vi "A170316-11_config.vi"() -> ()   [LabVIEW 2020]
uses:
  Global_Variable/Global.vi
  Database/Global1.vi
  <vilib>/Utility/config.llb/NI_LVConfig.lvlib
panel:
  in  "选项卡控件":enum32{"检具参数", "备用参数", "产品管理"}(tab)
  in  "检具选择":bool[](array[boolean])
  in  "删除":bool
  in  "确定":bool
  in  "添加":bool
  in  "退出":bool
  in  "更新":bool
  in  "产品型号":string(combo)
  in  "请输入添加的产品名称":string
  in  "请选择要删除的产品":string(combo)
  # "总成检验"
  # "检具1"
  # "检具2"
  # "检具3"
  # "检具4"
  # "检具5"
  # "检具6"
  # "检具7"
  # "检具8"
  # "检具9"
  # "检具10"
  # "检具11"
  # "检具12"
  # "检具13"
  # "检具14"
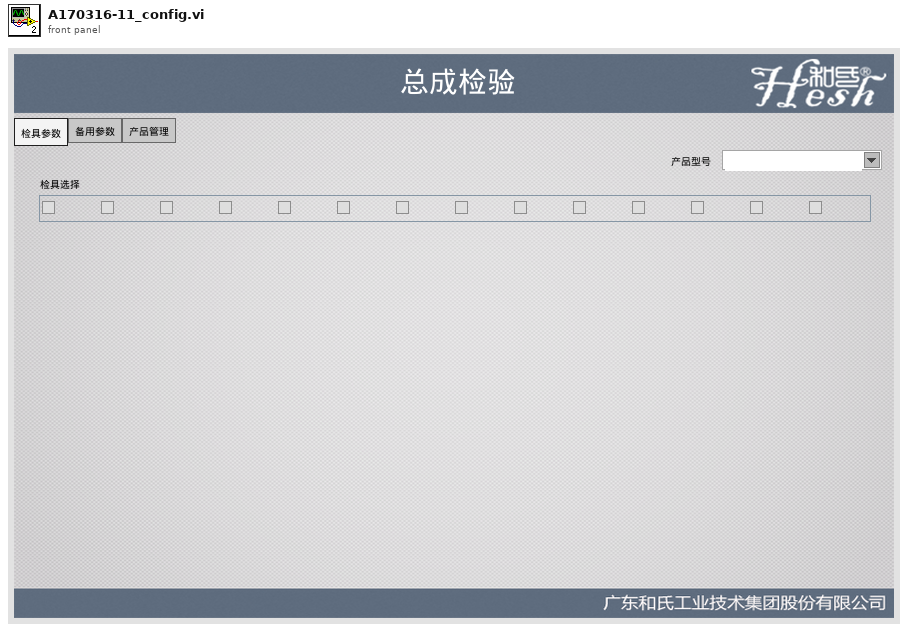
[diagram p1: front panel]
types:
  T1 = typedef "NI_LVConfig.lvlib/Config Data RefNum.ctl" = refnum<k1>
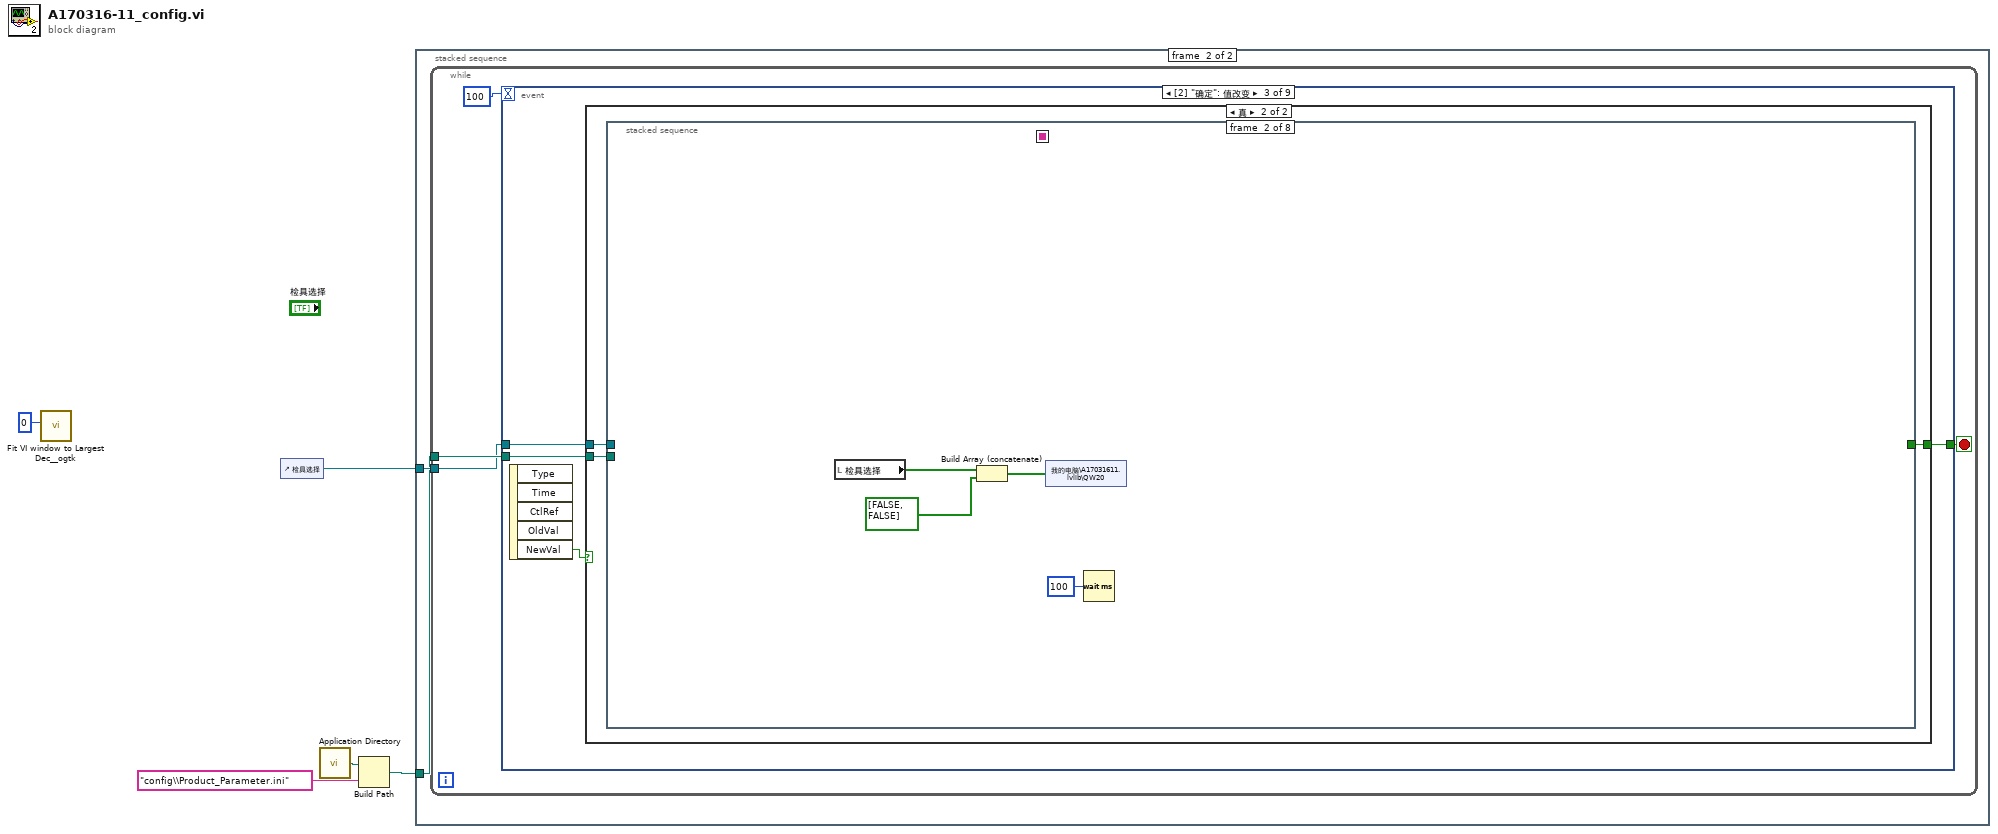
[diagram p0: block diagram]
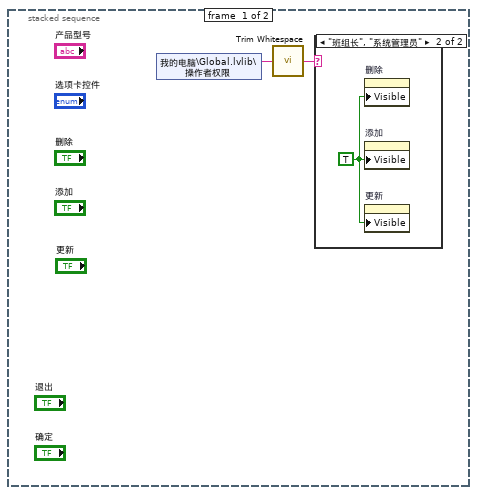
[diagram p2: hidden frame]
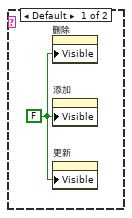
[diagram p3: hidden frame]
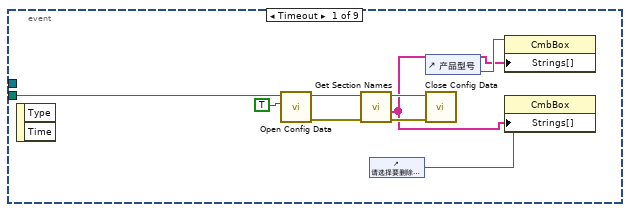
[diagram p4: hidden frame]
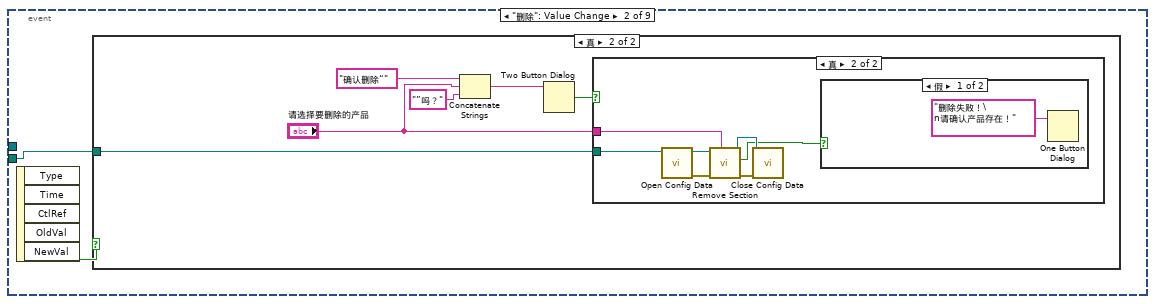
[diagram p5: hidden frame]
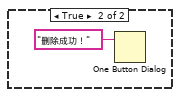
[diagram p8: hidden frame]
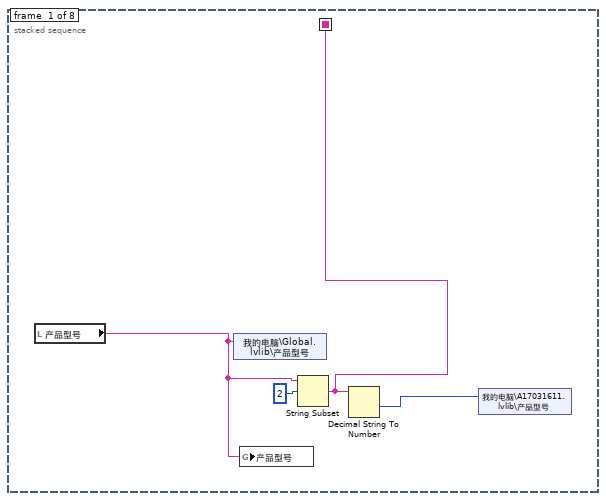
[diagram p10: hidden frame]
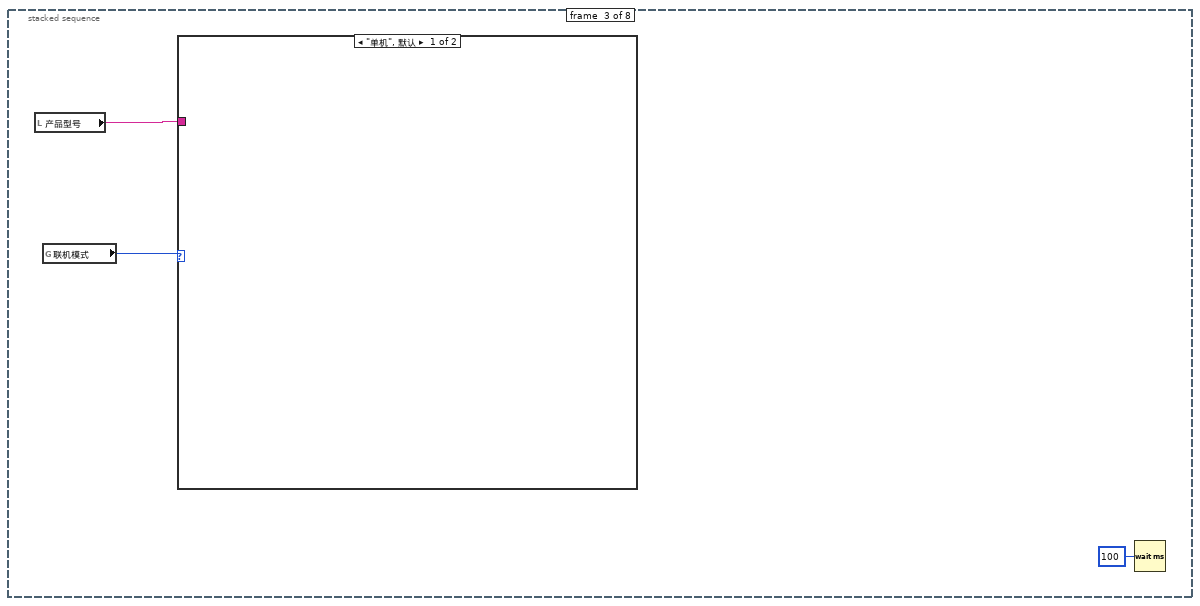
[diagram p11: hidden frame]
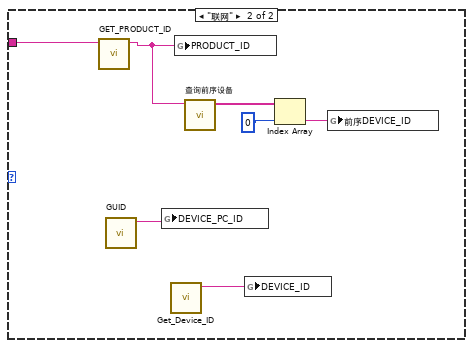
[diagram p12: hidden frame]
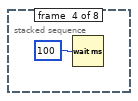
[diagram p13: hidden frame]
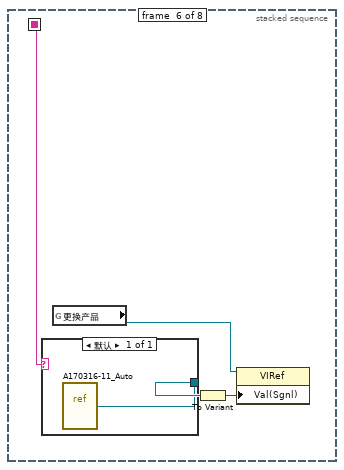
[diagram p15: hidden frame]
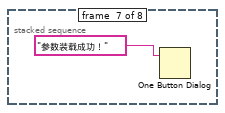
[diagram p16: hidden frame]
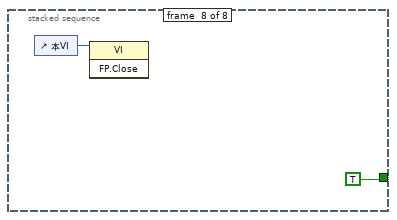
[diagram p17: hidden frame]
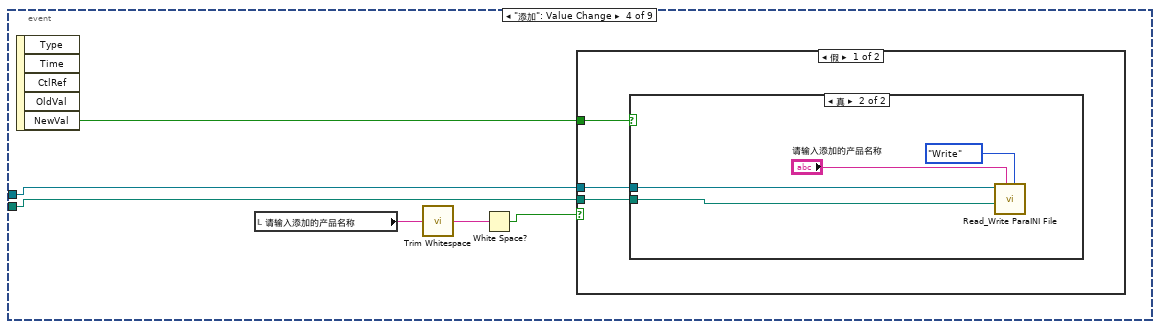
[diagram p18: hidden frame]
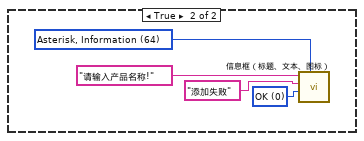
[diagram p20: hidden frame]
diagram:
  n1 = call <userlib>:"Fit VI window to Largest Dec__ogtk.vi"("border spacing (2 px)"=0) -> ()  [unwired: 5 in, 2 out]
  n2 = control-ref of="检具选择"() -> (w1:refnum<vi>)
  n3 = call <vilib>:"Application Directory.vi"() -> ("Application Directory"=w5:path)
  n4 = Build Path(base path=w5, name or relative path="config\\Product_Parameter.ini" ("名称或相对路径")) -> (appended path=w3:path)
  n5 = stacked-sequence {
    tunnel: w1 -> [_ w11]
    tunnel: w3 -> [_ w10]
    frame #0 {
      n6 = shared-variable "我的电脑\\Global.lvlib\\操作者权限"() -> (w7:string)  [unwired: 1 in, 1 out]
      n7 = call <vilib>:"Trim Whitespace.vi"("string"=w7) -> ("trimmed string"=w6:string)  [unwired: 1 in]
      n8 = case shown="\"班组长\", \"系统管理员\"" w6 {
        frame Default {
          w8 = FALSE ("可见")
          n9 = property on="删除" class="Bool (严格)"("Visible"=w8) -> ()  [unwired: 2 in, 2 out]
          n10 = property on="添加" class="Bool (严格)"("Visible"=w8) -> ()  [unwired: 2 in, 2 out]
          n11 = property on="更新" class="Bool (严格)"("Visible"=w8) -> ()  [unwired: 2 in, 2 out]
        }
        frame "班组长", "系统管理员" {
          w9 = TRUE ("可见")
          n12 = property on="删除" class="Bool (严格)"("Visible"=w9) -> ()  [unwired: 2 in, 2 out]
          n13 = property on="添加" class="Bool (严格)"("Visible"=w9) -> ()  [unwired: 2 in, 2 out]
          n14 = property on="更新" class="Bool (严格)"("Visible"=w9) -> ()  [unwired: 2 in, 2 out]
        }
      }
    }
    frame #1 {
      n15 = while {
        tunnel: w10 -> [w15]
        tunnel: w11 -> [w13]
        stop <- w14 stop-if-true
        n16 = event shown="[2] \"确定\": 值改变" {
          selector: _ -> [_ _ _ _ _ _ _ _ _]
          dyn-events: _ -> [_ _ _ _ _ _ _ _ _]
          timeout: 100 -> [_ _ _ _ _ _ _ _ _]
          tunnel: w15 -> [w19 w26 w42 w80 w95 _ w112 _ _]
          tunnel: [_ _ w44 _ _ TRUE _ _ TRUE] -> w14
          tunnel: w13 -> [_ _ w43 w81 w96 _ w111 _ _]
          event Timeout {
            n17 = event-data() -> ()  [unwired: 1 in, 2 out]
            n18 = call <vilib>:"Open Config Data.vi"("create file if necessary (T)"=TRUE, "configuration file path"=w19) -> ("error out"=w21:errorcluster, "refnum"=w20:T1)  [unwired: 7 in, 1 out]
            n19 = call <vilib>:"Get Section Names.vi"("error in (no error)"=w21, "refnum"=w20) -> ("error out"=w23:errorcluster, "section names"=w16:string[], "refnum out"=w22:T1)  [unwired: 7 in]
            n20 = control-ref of="请选择要删除的产品"() -> (w17:refnum<vi>)
            n21 = control-ref of="产品型号"() -> (w18:refnum<vi>)
            n22 = call <vilib>:"Close Config Data.vi"("error in (no error)"=w23, "refnum"=w22) -> ()  [unwired: 8 in, 2 out]
            n23 = property on="属性节点" class="CmbBox"(reference=w18, "Strings[]"=w16) -> ()  [unwired: 1 in, 2 out]
            n24 = property on="属性节点" class="CmbBox"(reference=w17, "Strings[]"=w16) -> ()  [unwired: 1 in, 2 out]
          }
          event "删除": Value Change {
            n25 = event-data() -> ("NewVal"=w25:bool)  [unwired: 1 in, 4 out]
            n26 = case shown="真" w25 {
              tunnel: w26 -> [_ w28]
              frame False {
              }
              frame True {
                n27 = Concatenate Strings("确认删除“", "请选择要删除的产品", "”吗？") -> (w30:string)
                n28 = Two Button Dialog(message=w30) -> (T button?=w29:bool)  [unwired: 2 in]
                n29 = case shown="真" w29 {
                  tunnel: w28 -> [_ w34]
                  tunnel: "请选择要删除的产品" -> [_ w33]
                  frame False {
                  }
                  frame True {
                    n30 = call <vilib>:"Open Config Data.vi"("configuration file path"=w34) -> ("error out"=w36:errorcluster, "refnum"=w39:T1)  [unwired: 8 in, 1 out]
                    n31 = call <vilib>:"Remove Section.vi"("section"=w33, "error in (no error)"=w36, "refnum"=w39) -> ("error out"=w38:errorcluster, "section exists?"=w35:bool, "refnum out"=w37:T1)  [unwired: 6 in]
                    n32 = call <vilib>:"Close Config Data.vi"("error in (no error)"=w38, "refnum"=w37) -> ()  [unwired: 8 in, 2 out]
                    n33 = case shown="假" w35 {
                      frame False {
                        n34 = One Button Dialog(message="删除失败！\n请确认产品存在！" ("消息")) -> ()  [unwired: 1 in, 1 out]
                      }
                      frame True {
                        n35 = One Button Dialog(message="删除成功！" ("消息")) -> ()  [unwired: 1 in, 1 out]
                      }
                    }
                  }
                }
              }
            }
          }
          event "确定": Value Change {
            n36 = event-data() -> ("NewVal"=w45:bool)  [unwired: 1 in, 4 out]
            n37 = case shown="真" w45 {
              tunnel: [_ w48] -> w44
              tunnel: w43 -> [_ w47]
              tunnel: w42 -> [_ w46]
              frame False {
              }
              frame True {
                n38 = stacked-sequence {
                  seq-local: [w52 _ _ _ _ _ _ _] -> [_ _ _ _ _ w71 _ _]
                  tunnel: [_ _ _ _ _ _ _ TRUE] -> w48
                  tunnel: w47 -> [_ _ _ _ _ _ _ _]
                  tunnel: w46 -> [_ _ _ _ _ _ _ _]
                  frame #0 {
                    n39 = local read "产品型号"() -> (w49:string)
                    n40 = shared-variable "我的电脑\\Global.lvlib\\产品型号"(w49) -> ()  [unwired: 1 in, 1 out]
                    n41 = global write "Global.vi" "产品型号"(w49) -> ()
                    n42 = String Subset(string=w49, offset (0)=u16 2 ("偏移量(0)")) -> (substring=w52:string)  [unwired: 1 in]
                    n43 = Decimal String To Number(string=w52) -> (number=w50:i32)  [unwired: 2 in, 1 out]
                    n44 = shared-variable "我的电脑\\A17031611.lvlib\\产品型号"(w50) -> ()  [unwired: 1 in, 1 out]
                  }
                  frame #1 {
                    n45 = local read "检具选择"() -> (w55:bool[])
                    n46 = Build Array (concatenate)(w55, bool[] [FALSE, FALSE] ("数组")) -> (w54:bool[])
                    n47 = shared-variable "我的电脑\\A17031611.lvlib\\QW20"(w54) -> ()  [unwired: 1 in, 1 out]
                    n48 = Wait (ms)(milliseconds to wait=u32 100) -> ()  [unwired: 1 out]
                  }
                  frame #2 {
                    n49 = local read "产品型号"() -> (w58:string)
                    n50 = global read "Global1.vi" "联机模式"() -> (w57:enum16{"单机", "联网"})
                    n51 = case shown="\"单机\", 默认" w57 {
                      tunnel: w58 -> [_ w60]
                      frame "单机", Default {
                      }
                      frame "联网" {
                        n52 = call "GET_PRODUCT_ID.vi"("PRODFUCT_NAME"=w60) -> ("PRODUCT_ID"=w65:string)  [unwired: 10 in]
                        n53 = call "GUID.vi"() -> ("trimmed string"=w66:string)  [unwired: 11 in]
                        n54 = global write "Global1.vi" "DEVICE_PC_ID"(w66) -> ()
                        n55 = call "Get_Device_ID.vi"() -> ("Device_ID"=w61:string)  [unwired: 10 in, 1 out]
                        n56 = global write "Global1.vi" "PRODUCT_ID"(w65) -> ()
                        n57 = call "查询前序设备.vi"("PRODUCT_ID"=w65) -> ("前序工位"=w64:string[])  [unwired: 10 in]
                        n58 = global write "Global1.vi" "DEVICE_ID"(w61) -> ()
                        n59 = Index Array(array=w64, index=0 ("索引")) -> (element=w62:string)
                        n60 = global write "Global1.vi" "前序DEVICE_ID"(w62) -> ()
                      }
                    }
                    n61 = Wait (ms)(milliseconds to wait=u32 100) -> ()  [unwired: 1 out]
                  }
                  frame #3 {
                    n62 = Wait (ms)(milliseconds to wait=u32 100) -> ()  [unwired: 1 out]
                  }
                  frame #4 {
                  }
                  frame #5 {
                    n63 = case shown="默认" w71 {
                      tunnel: [w72] -> w68
                      frame 默认 {
                        n64 = vi-ref "A170316-11_Auto.vi"() -> (w72:refnum<vi>)
                      }
                    }
                    n65 = global read "Global.vi" "更换产品"() -> (w70:refnum<vi>)
                    n66 = To Variant(anything=w68) -> (Variant=w69:variant)
                    n67 = property class="VIRef"(reference=w70, "Val(Sgnl)"=w69) -> ()  [unwired: 1 in, 2 out]
                  }
                  frame #6 {
                    n68 = One Button Dialog(message="参数装载成功！" ("消息")) -> ()  [unwired: 1 in, 1 out]
                  }
                  frame #7 {
                    n69 = control-ref of="本VI"() -> (w74:refnum<vi>)
                    n70 = invoke class="VI" method="FP.Close"(reference=w74) -> ()  [unwired: 2 in, 3 out]
                  }
                }
              }
            }
          }
          event "添加": Value Change {
            n71 = event-data() -> ("NewVal"=w79:bool)  [unwired: 1 in, 4 out]
            n72 = local read "请输入添加的产品名称"() -> (w78:string)
            n73 = call <vilib>:"Trim Whitespace.vi"("string"=w78) -> ("trimmed string"=w76:string)  [unwired: 1 in]
            n74 = White Space?(1:w76) -> (0:w77:bool)
            n75 = case shown="假" w77 {
              tunnel: w81 -> [w84 _]
              tunnel: w80 -> [w83 _]
              tunnel: w79 -> [w82 _]
              frame False {
                n76 = case shown="真" w82 {
                  tunnel: w84 -> [_ w88]
                  tunnel: w83 -> [_ w87]
                  frame False {
                  }
                  frame True {
                    n77 = call "Read_Write ParaINI File.vi"("Mode"=enum16{"Read", "Write"}."Write", "Section"="请输入添加的产品名称", "Filepath"=w87, "Ctl Refnum"=w88) -> ()  [unwired: 7 in, 1 out]
                  }
                }
              }
              frame True {
                w89 = 64 items=["None"=0, "Hand, Error, Stop"=16, "Question"=32, "Exclamation, Warning"=48, "Asterisk, Information"=64] ("icon")
                w90 = 0 items=["OK", "OKCancel", "AbortRetryIgnore", "YesNoCancel", "YesNo", "RetryCancel"] ("buttons")
                n78 = call "信息框（标题、文本、图标）.vi"("icon"=w89, "buttons"=w90, "caption"="添加失败", "text"="请输入产品名称!") -> ()  [unwired: 6 in, 2 out]
              }
            }
          }
          event "产品型号": Value Change {
            n79 = event-data() -> ("CtlRef"=w94:refnum<vi>, "NewVal"=w93:string)  [unwired: 1 in, 3 out]
            n80 = stacked-sequence {
              tunnel: w96 -> [_ w105]
              tunnel: w95 -> [_ w104]
              tunnel: w94 -> [w98 _]
              tunnel: w93 -> [w97 _]
              frame #0 {
                n81 = stacked-sequence {
                  tunnel: w98 -> [_ w100]
                  tunnel: w97 -> [_ w101]
                  frame #0 {
                    n82 = control-ref of="This VI"() -> (w99:refnum<vi>)
                    n83 = invoke class="VI" method="Default Vals.Reinit All"(reference=w99) -> ()  [unwired: 2 in, 3 out]
                  }
                  frame #1 {
                    n84 = property class="CmbBox"(reference=w100, "Value"=w101) -> ()  [unwired: 1 in, 2 out]
                  }
                }
              }
              frame #1 {
                n85 = local read "产品型号"() -> (w102:string)
                n86 = call "Read_Write ParaINI File.vi"("Mode"=enum16{"Read", "Write"}."Read", "Section"=w102, "Filepath"=w104, "Ctl Refnum"=w105) -> ()  [unwired: 7 in, 1 out]
              }
            }
          }
          event "退出": Value Change {
            n87 = event-data() -> ()  [unwired: 1 in, 5 out]
            n88 = control-ref of="本VI"() -> (w108:refnum<vi>)
            n89 = invoke class="VI" method="FP.Close"(reference=w108) -> (reference out=w106:refnum<vi>, error out=w107:errorcluster)  [unwired: 2 in, 1 out]
            n90 = Close Reference(reference=w106, error in (no error)=w107) -> ()  [unwired: 1 out]
          }
          event "更新": Value Change {
            n91 = event-data() -> ("NewVal"=w110:bool)  [unwired: 1 in, 4 out]
            n92 = case shown="真" w110 {
              tunnel: w112 -> [_ w117]
              tunnel: w111 -> [_ w116]
              frame False {
              }
              frame True {
                n93 = local read "产品型号"() -> (w114:string)
                n94 = call "Read_Write ParaINI File.vi"("Mode"=enum16{"Read", "Write"}."Write", "Section"=w114, "Filepath"=w117, "Ctl Refnum"=w116) -> ("error out"=w115:errorcluster)  [unwired: 7 in]
                n95 = case shown="无错误" w115 {
                  frame No Error {
                    n96 = call "浮动通知.vi"("通知内容"="更新成功！") -> ()  [unwired: 11 in]
                  }
                  frame Error {
                    n97 = call "浮动通知.vi"("通知内容"="更新失败！") -> ()  [unwired: 11 in]
                  }
                }
              }
            }
          }
          event "请输入添加的产品名称": Value Change {
            n98 = event-data() -> ("NewVal"=w122:string)  [unwired: 1 in, 4 out]
            n99 = control-ref of="产品型号"() -> (w120:refnum<vi>)
            n100 = property on="属性节点" class="CmbBox"(reference=w120) -> ("Strings[]"=w121:string[])  [unwired: 1 in, 2 out]
            n101 = for {
              tunnel: w122 -> [w123]
              tunnel: w121 -> [w124] mode=indexing
              n102 = Equal?(x=w123, y=w124) -> (x = y?=w125:bool)
              n103 = case shown="真" w125 {
                tunnel: w123 -> [_ w126]
                frame False {
                }
                frame True {
                  n104 = stacked-sequence {
                    tunnel: w126 -> [w132 _]
                    frame #0 {
                      w127 = 64 items=["None"=0, "Hand, Error, Stop"=16, "Question"=32, "Exclamation, Warning"=48, "Asterisk, Information"=64] ("icon")
                      w128 = 0 items=["OK", "OKCancel", "AbortRetryIgnore", "YesNoCancel", "YesNo", "RetryCancel"] ("buttons")
                      n105 = Concatenate Strings("已经存在产品”" ("text"), w132, "“\n请勿重复添加！" ("字符串")) -> (w130:string)
                      n106 = call "信息框（标题、文本、图标）.vi"("icon"=w127, "buttons"=w128, "caption"="产品重复", "text"=w130) -> ()  [unwired: 6 in, 2 out]
                    }
                    frame #1 {
                      n107 = local write "请输入添加的产品名称"("" ("请输入添加的产品名称")) -> ()
                    }
                  }
                }
              }
            }
          }
          event Panel Close {
            n108 = event-data() -> ()  [unwired: 1 in, 3 out]
          }
        }
      }
    }
  }
